vi "Update Table.vi"(8 "error in (no error)":errorcluster, 10 "Table":refnum<class "Basic Table.lvclass">, 11 "Form Model in":refnum<class "Form Model.lvclass">) -> (0 "error out":errorcluster, 3 "Form Model out":refnum<class "Form Model.lvclass">)   [LabVIEW 2020, in "Form Model.lvlib" / "Form Model.lvclass"]
uses:
  Form Model.lvclass
  Database OOP/Table Libraries/Basic Table/Basic Table Class/Basic Table.lvclass
  Form Model.lvclass/Form Model.ctl
  Panel Form Controller Messages/Update Table Msg/Update Table Msg.lvclass/Update Table Msg.ctl
  <vilib>/ActorFramework/Message Enqueuer/Message Enqueuer.lvclass/Message Enqueuer.ctl
  <vilib>/ActorFramework/Message Enqueuer/Enqueue.vi
  Panel Form Controller Messages/Update Table Msg/Update Table Msg.lvclass
  C:/Program Files (x86)/National Instruments/LabVIEW 2020/vi.lib/ActorFramework/Message/Message.lvclass
  <vilib>/ActorFramework/Message Priority Queue/Priority Enqueue.vi
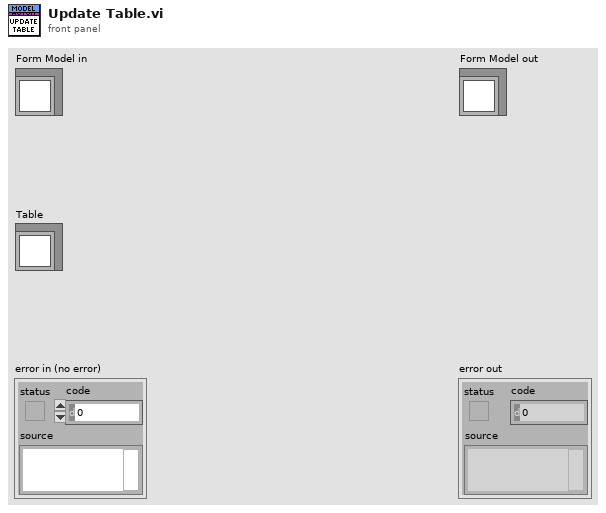
[diagram p1: front panel]
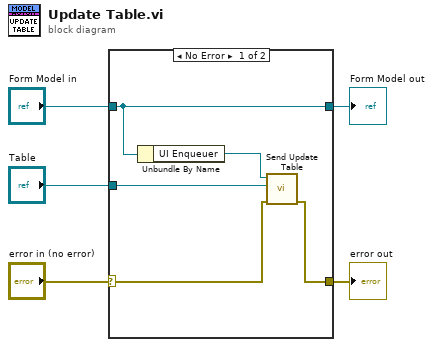
[diagram p0: block diagram]
diagram:
  n1 = case shown="No Error" "error in (no error)" {
    selector: "error in (no error)" -> [w9 w12]
    tunnel: [w8 w12] -> w4
    tunnel: "Form Model in" -> [w6 w11]
    tunnel: [w6 w11] -> w2
    tunnel: "Table" -> [w10 _]
    frame No Error {
      n2 = Unbundle By Name(w6) -> ("UI Enqueuer"=w7:refnum<class "Message Enqueuer.lvclass">)
      n3 = call "Send Update Table.vi"("error in (no error)"=w9, "Table"=w10, "Message Enqueuer"=w7) -> ("error out"=w8:errorcluster)  [unwired: 7 in, 1 out]
    }
    frame Error {
    }
  }
  "error out" <- w4
  "Form Model out" <- w2
